vi "Configure Linear Mode Sweep.vi"(0 "VISA resource name":refnum<visa-resource-name>, 1 "Source Mode  (0: Voltage)":u16(ring) items=["Voltage", "Current"], 2 "Sweep Points":T1={"Start "=1.0, "Stop "=0.0, "Number of Points (5)"=5}, 3 "Delay (0)":dbl, 4 "Count (1)":i32=1, 5 "error in (no error)":errorcluster, 6 "Fail Abort (T:ON)":bool=TRUE, 7 "Range Type  (0: Best Fixed Range)":u16(ring)=1 items=["Most Sensitive Source Range", "Best Fixed Range", "Present Source Range"], 8 "Dual (T:OFF)":bool, 9 "Buffer Name (defbuffer1)":string="defbuffer1") -> (14 "VISA resource name out":refnum<visa-resource-name>, 19 "error out":errorcluster)   [LabVIEW 2015, in "Keithley 2450.lvlib"]
doc: "This sets up a linear sweep for a set number of measurement points."
uses:
  <instrlib>/Keithley 2450/Keithley 2450.lvlib
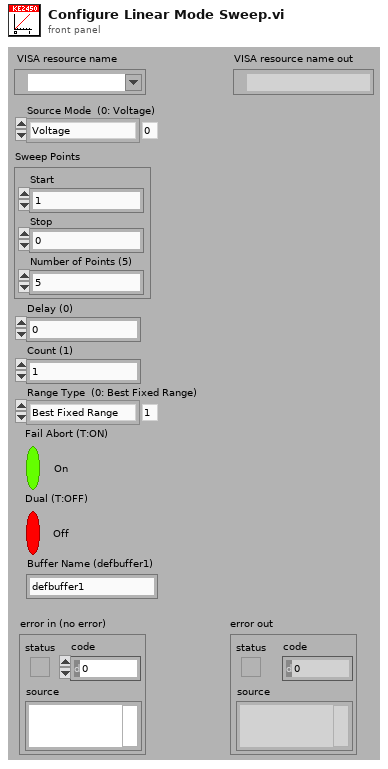
[diagram p1: front panel]
types:
  T1 = cluster{"Start ":dbl, "Stop ":dbl, "Number of Points (5)":u32}
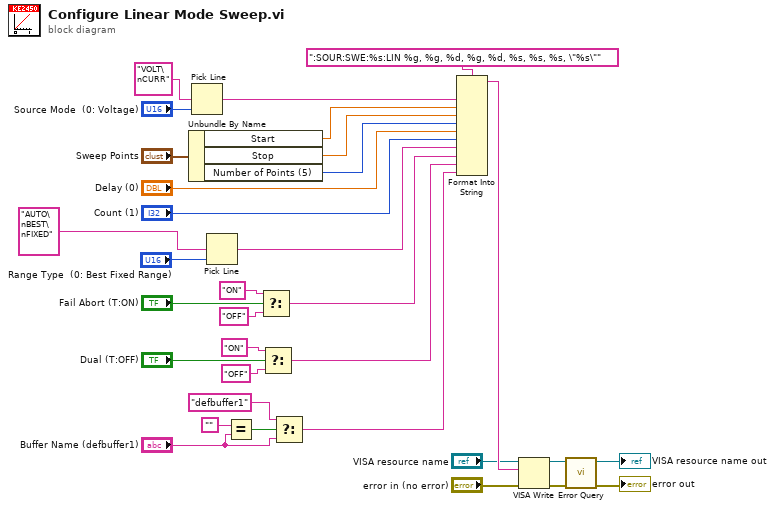
[diagram p0: block diagram]
diagram:
  n1 = Unbundle By Name("Sweep Points") -> ("Start"=w24:dbl, "Stop"=w23:dbl, "Number of Points (5)"=w22:u32)
  n2 = Pick Line(multi-line string="VOLT\nCURR" ("string (\"\")"), line index="Source Mode  (0: Voltage)") -> (output string=w30:string)  [unwired: 1 out]
  n3 = Pick Line(multi-line string="AUTO\nBEST\nFIXED" ("string (\"\")"), line index="Range Type  (0: Best Fixed Range)") -> (output string=w3:string)  [unwired: 1 out]
  n4 = Equal?(x="", y="Buffer Name (defbuffer1)") -> (x = y?=w9:bool)
  n5 = Select(t="ON" ("Buffer Name (defbuffer1)"), s="Fail Abort (T:ON)", f="OFF" ("Buffer Name (defbuffer1)")) -> (s? t:f=w17:string)
  n6 = Select(t="ON" ("Buffer Name (defbuffer1)"), s="Dual (T:OFF)", f="OFF" ("Buffer Name (defbuffer1)")) -> (s? t:f=w11:string)
  n7 = Select(t="defbuffer1", s=w9, f="Buffer Name (defbuffer1)") -> (s? t:f=w7:string)
  n8 = Format Into String(format string=":SOUR:SWE:%s:LIN %g, %g, %d, %g, %d, %s, %s, %s, \"%s\"", w30, w24, w23, w22, "Delay (0)", "Count (1)", w3, w17, w11, w7) -> (resulting string=w18:string)  [unwired: 2 in, 1 out]
  n9 = VISA Write(VISA resource name="VISA resource name", write buffer=w18, error in (no error)="error in (no error)") -> (VISA resource name out=w29:refnum<visa-resource-name>, error out=w28:errorcluster)  [unwired: 1 out]
  n10 = call <instrlib>:"Error Query.vi"("error in (no error)"=w28, "VISA resource name"=w29) -> ("error out"=→"error out":errorcluster, "VISA resource name out"=→"VISA resource name out":refnum<visa-resource-name>)  [unwired: 8 out]
